vi "Disconnect.vi"(8 "error in (no error)":errorcluster, 10 "Stream:Connection":refnum<class "Connection.lvclass">, 11 "Manager in":refnum<class "Manager.lvclass">) -> (0 "error out":errorcluster, 1 "Exists":bool, 2 "Endpoint":refnum<class "Endpoint.lvclass">, 3 "Manager out":refnum<class "Manager.lvclass">)   [LabVIEW 2020, in "Stream-Simple-Msg.lvlib" / "Manager.lvclass"]
uses:
  Manager.lvclass
  <vilib>/IlluminatedG/lv-stream/Connection/Connection.lvclass
  C:/Program Files (x86)/National Instruments/LabVIEW 2020/vi.lib/IlluminatedG/lv-stream/Endpoint/Endpoint.lvclass
  Endpoint/Endpoint.lvclass
  Manager.lvclass/Manager.ctl
  <vilib>/IlluminatedG/lv-stream/Endpoint/Endpoint.lvclass
  <vilib>/IlluminatedG/lv-stream/URI/URI.lvclass
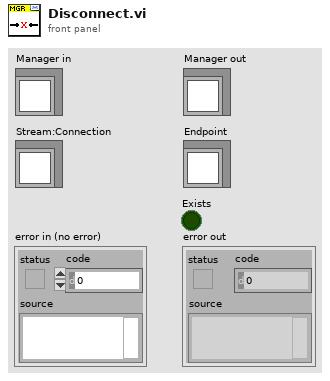
[diagram p1: front panel]
types:
  T1 = typedef "Stream-Simple-Msg.lvlib/Manager.lvclass/Ref Data.ctl" = cluster{"Message Callbacks":map{string, T2[]}, "Endpoints":map{string, T3}, "Stream Endpoints":refnum<class "Endpoint.lvclass">[], "State Callbacks":T5[], "Stream Formats":T4[]}
  T2 = typedef "Stream-Simple-Msg.lvlib/Manager.lvclass/Callback.ctl" = cluster{"VI":refnum<vi>, "Owner":refnum<class>}
  T3 = typedef "Stream-Simple-Msg.lvlib/Manager.lvclass/Mapped Endpoint.ctl" = cluster{"Msg Endpoint":refnum<class "Endpoint.lvclass">, "Format":T4}
  T4 = typedef "Stream-Simple-Msg.lvlib/Format.ctl" = enum16{"LabVIEW Binary", "JSON"}
  T5 = typedef "Stream-Simple-Msg.lvlib/Manager.lvclass/State Callback.ctl" = cluster{"Owner":refnum<class>, "VI":refnum<vi>, "Context":variant}
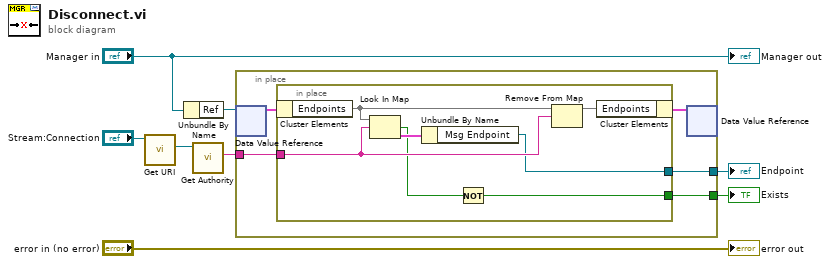
[diagram p0: block diagram]
diagram:
  n1 = call <vilib>:"Get URI.vi"("Endpoint in"="Stream:Connection") -> ("URI"=w4:refnum<class "URI.lvclass">)  [unwired: 8 in, 2 out]
  n2 = Unbundle By Name("Manager in") -> ("Ref"=w6:refnum<data-value>)
  n3 = call <vilib>:"Get Authority.vi"("URI in"=w4) -> ("Authority"=w3:string)  [unwired: 8 in, 2 out]
  n4 = in-place {
    in-place-border: w3 -> [w12]
    in-place-border: [w10] -> w2
    in-place-border: [w9] -> w1
    n5 = in-place-dvr #1(w6) -> (w13:T1)  [unwired: 1 out]
    n6 = in-place {
      in-place-border: w12 -> [w18]
      in-place-border: [w16] -> w10
      in-place-border: [w14] -> w9
      n7 = in-place-cluster #2(w13) -> ("Endpoints"=w20:map{string, T3})
      n8 = Look In Map(map=w20, key=w18) -> (key not found?=w15:bool, value=w17:T3)  [unwired: 1 in]
      n9 = Unbundle By Name(w17) -> ("Msg Endpoint"=w16:refnum<class "Endpoint.lvclass">)
      n10 = Not(x=w15) -> (.not. x?=w14:bool)
      n11 = Remove From Map(10:w18, 11:w20) -> (3:w19:map{string, T3})  [unwired: 2 out]
      n12 = in-place-cluster #2("Endpoints"=w19) -> (w11:T1)
    }
    n13 = in-place-dvr #1(w11) -> ()  [unwired: 2 out]
  }
  "Endpoint" <- w2
  "Exists" <- w1
  "error out" <- "error in (no error)"
  "Manager out" <- "Manager in"
